vi "Get_Step.vi"(8 "error in (no error)":errorcluster, 11 "Lifter_motor in":refnum<class "Lifter_motor.lvclass">) -> (0 "error out":errorcluster, 2 "Step Count":i32, 3 "Lifter_motor out":refnum<class "Lifter_motor.lvclass">)   [LabVIEW 2019, in "Lifter_motor.lvclass"]
uses:
  Lifter_motor.lvclass
  Lifter_motor.lvclass/Lifter_motor.ctl
  TCP Class/LifterTCP.lvclass
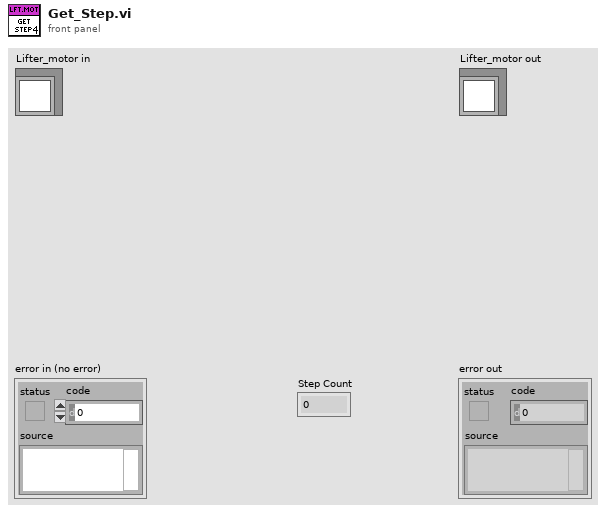
[diagram p1: front panel]
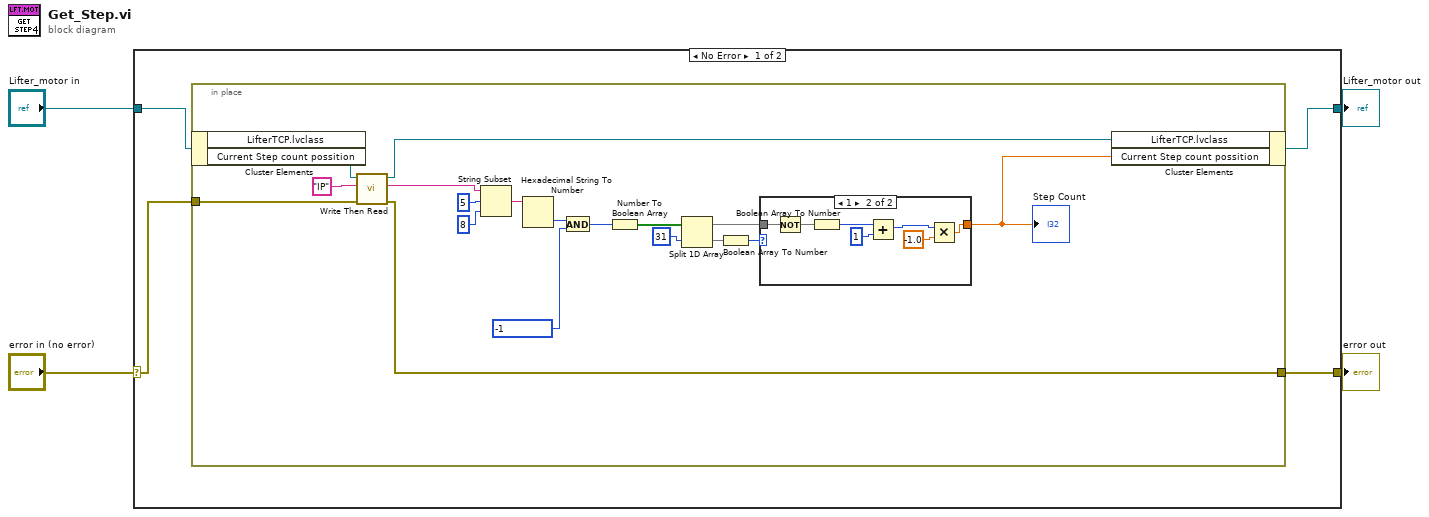
[diagram p0: block diagram]
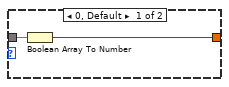
[diagram p2: hidden frame]
diagram:
  n1 = case shown="No Error" "error in (no error)" {
    selector: "error in (no error)" -> [w6 w37]
    tunnel: [w5 w37] -> w3
    tunnel: [w7 w36] -> w1
    tunnel: "Lifter_motor in" -> [w8 w36]
    frame No Error {
      n2 = in-place {
        in-place-border: w6 -> [w25]
        in-place-border: [w11] -> w5
        n3 = in-place-cluster #1(w8) -> ("LifterTCP.lvclass"=w26:refnum<class "LifterTCP.lvclass">)  [unwired: 1 out]
        n4 = call "Write Then Read.vi"("error in (no error)"=w25, "Parameter 1"="IP", "LifterTCP in"=w26) -> ("error out"=w11:errorcluster, "Read Data"=w12:string, "LifterTCP out"=w24:refnum<class "LifterTCP.lvclass">)  [unwired: 6 in]
        n5 = String Subset(string=w12, offset (0)=5, length (rest)=8 ("length (rest)")) -> (substring=w23:string)
        n6 = Hexadecimal String To Number(string=w23) -> (number=w20:u32)  [unwired: 2 in, 1 out]
        n7 = And ("Just the \n12 bits")(x=w20, y=-1 ("number")) -> (x .and. y?=w14:u32)
        n8 = Number To Boolean Array(number=w14) -> (Boolean array=w15:bool[])
        n9 = Split 1D Array(array=w15, index=31) -> (first subarray=w18:bool[], second subarray=w16:bool[])
        n10 = Boolean Array To Number(Boolean array=w16) -> (number=w19:u32)
        n11 = case shown="1" w19 {
          tunnel: w18 -> [w28 w35]
          tunnel: [w27 w30] -> w9
          frame 0, Default {
            n12 = Boolean Array To Number(Boolean array=w28) -> (number=w27:u32)
          }
          frame 1 {
            n13 = Not(x=w35) -> (.not. x?=w34:bool[])
            n14 = Boolean Array To Number(Boolean array=w34) -> (number=w32:u32)
            n15 = Add(x=w32, y=u32 1) -> (x+y=w29:u32)
            n16 = Multiply(x=w29, y=-1.0) -> (x*y=w30:dbl)
          }
        }
        "Step Count" <- w9
        n17 = in-place-cluster #1("LifterTCP.lvclass"=w24, "Current Step count possition"=w9) -> (w7:refnum<class "Lifter_motor.lvclass">)
      }
    }
    frame Error {
    }
  }
  "error out" <- w3
  "Lifter_motor out" <- w1
